vi "S Parameter Pre-Processing.vi"(6 "Username (\"\")":string, 7 "Fields In":T1[](array[typedef]), 8 "error in (no error)":errorcluster, 10 "Test Configuration (\"\")":string, 11 "Test_ID (\"\")":string) -> (0 "error out":errorcluster, 1 "Files Found?":bool, 2 "New Test Configuration":string, 3 "Dup Test_ID":string, 5 "Fields Out":T1[](array[typedef]))   [LabVIEW 2011]
uses:
  typedefs/Field Record.ctl
  typedefs/Field DataTypes.ctl
  typedefs/Field NextItem.ctl
  typedefs/Field System Fields.ctl
  TypeDefs/SP Limit Point.ctl
  LIB/S Parameter Version.vi
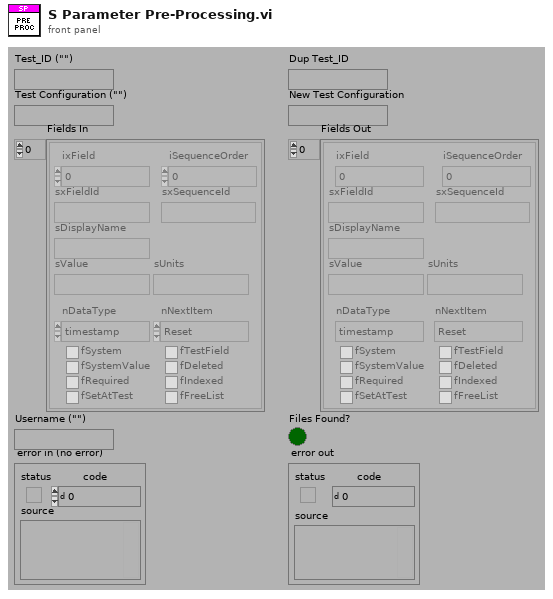
[diagram p1: front panel]
types:
  T1 = typedef "Field Record.ctl" = cluster{"ixField":i32, "iSequenceOrder":i32, "sxFieldId":string, "sxSequenceId":string, "sDisplayName":string, "sValue":string, "sUnits":string, "nDataType":T2, "nNextItem":T3, "fSystem":bool, "fSystemValue":bool, "fRequired":bool, "fSetAtTest":bool, "fTestField":bool, "fDeleted":bool, "fIndexed":bool, "fFreeList":bool}
  T2 = typedef "Field DataTypes.ctl" = enum32{"text", "numeric", "list", "timestamp", "boolean"}
  T3 = typedef "Field NextItem.ctl" = enum32{"Reset", "Retain", "Auto-Increment"}
  T4 = cluster{"Ref Limit":bool, "Ref Type":bool, "Model":bool, "Serial":bool, "Run Type":bool, "Run":bool, "Field":bool, "Field Value":bool}
  T5 = typedef "Field System Fields.ctl" = enum32{"Company", "End_Timestamp", "Model_Number", "Operator", "Serial_Number", "Start_Timestamp", "Step_Number", "Step_Tag", "Test_Run", "Test_Sequence", "Test_Station", "Test_Station_Name", "Test_Status", "Test_Type", "Test_Version", "Spartan_Version_Created", "Spartan_Version_Current"}
  T6 = typedef "SP Limit Point.ctl" = cluster{"Frequency":dbl, "Value":dbl, "X":dbl, "Y":dbl, "Connected":bool}
  T7 = typedef "SP Test Parameters.ctl" = cluster{"Stimulus":T8, "Measurement":T11, "De-Embed":T14, "Display":T17, "Limits":T24[], "Filter Limits":T28[]}
  T8 = typedef "SP Stimulus Parameters.ctl" = cluster{"Use Instrument Settings":bool, "Blank Frequencies":bool, "Sweep Type":enum32{"Linear", "Logarithmic", "List", "Power", "CW"}, "Sweep":cluster{"Fstart":dbl, "Fstop":dbl, "Units":T9, "Points":i32}, "Power (dBm)":dbl, "IFBW (Hz)":dbl, "Sweep Time (s)":dbl, "Calibration":T10}
  T9 = typedef "SP Frequency Units.ctl" = enum16{"Hz", "kHz", "MHz", "GHz", "Points"}
  T10 = typedef "SP Calibration State.ctl" = cluster{"State":bool, "String":string}
  T11 = typedef "SP Measurement.ctl" = cluster{"Auto Select":bool, "Data Source":enum16{"VNA", "Data File"}, "Ports":i8, "Parameters":T12[]}
  T12 = typedef "SP Parameters.ctl" = cluster{"Channel":i8, "Parameter":T13}
  T13 = typedef "SP Parameter.ctl" = cluster{"Stimulus Port":i8, "Response Port":i8}
  T14 = typedef "SP De-Embed.ctl" = cluster{"De-Embed":bool, "Adapters":T15[]}
  T15 = typedef "SP Adapter.ctl" = cluster{"Port":i8, "Order":i8, "Model Number":string, "Serial Number":string, "SP Data":T16, "Run Type":enum16{"Most Recent", "Run #", "Match Field"}, "Run":i32, "Field":string, "Field Value":string}
  T16 = typedef "SP Data.ctl" = cluster{"F0":dbl, "dF":dbl, "Data":cdb[][]}
  T17 = typedef "SP Display Parameters.ctl" = cluster{"Lock Control":bool, "Retain Settings":bool, "Formatted Data":bool, "Plot Orientation":enum32{"Single", "Dual", "Quad"}, "Plot Controls":T18[]}
  T18 = typedef "SP Display Plot Controls Cluster.ctl" = cluster{"Trace Orientation":enum32{"Overlay", "Split"}, "Frequency":cluster{"Change Frequency":bool, "Start":dbl, "Stop":dbl, "Units":T9}, "Markers":T19[], "Traces":T21[]}
  T19 = typedef "SP Marker Cluster.ctl" = cluster{"Type":T20, "Frequency (MHz)":dbl}
  T20 = typedef "SP Marker Type.ctl" = enum16{"Frequency", "Trace Maximum", "Trace Minimum", "Limit Maximum", "Limit Minimum"}
  T21 = typedef "SP Display Trace Controls.ctl" = cluster{"Trace On":bool, "Measure":i32, "Format":T22, "Autoscale":bool, "Reference":dbl, "\nRefUnit":string, "Position":dbl, "Scale":dbl, "ScaleUnit":string, "LimitOn":bool, "LimitFill":bool, "Display Data":T23, "Show Markers":bool, "SXX":string}
  T22 = typedef "SP Display Format.ctl" = i32
  T23 = typedef "SP Display Data.ctl" = u16
  T24 = typedef "SP Limit.ctl" = cluster{"Parameter":T13, "Format":T25, "Limit Type":T26, "Points":T6[], "Referential Limit":T27, "Limit #":i8}
  T25 = typedef "SP Format.ctl" = enum16{"Log Mag", "Lin Mag", "SWR", "Phase", "Expanded Phase", "Delay", "Insertion Loss", "Isolation", "Return Loss"}
  T26 = typedef "SP Limit Type.ctl" = enum16{"Upper", "Lower", "Delta", "Filter", "Referential"}
  T27 = typedef "Test Referential Limit.ctl" = cluster{"Ref Limit":bool, "Ref Type":enum16{"Current", "Specify"}, "Model":string, "Serial":string, "Run Type":enum16{"Most Recent", "Run #", "Match Field"}, "Run":i32, "Field":string, "Field Value":string}
  T28 = typedef "SP Filter.ctl" = cluster{"Limit #":i8, "Parameter":T13, "Format":T25, "Filter Type":T29, "Passband":T30, "Ripple":T32, "Attenuation Points":T33[], "Skirt Points":T35[]}
  T29 = typedef "SP Filter Type.ctl" = enum16{"Lowpass", "Highpass", "Bandpass", "Bandstop"}
  T30 = typedef "SP Filter Passband.ctl" = cluster{"Start/Center":dbl, "Stop/Span":dbl, "Units":T9, "Freq Format":T31, "Bandwidth Attn":dbl, "Passband Limit":bool}
  T31 = typedef "SP Frequency Format.ctl" = enum16{"Start/Stop", "Center/Span"}
  T32 = typedef "SP Filter Ripple.ctl" = cluster{"Ripple Limit":bool, "Window On":bool, "Ripple":dbl, "Window":dbl, "Units":T9}
  T33 = typedef "SP Attenuation Point.ctl" = cluster{"Attenuation":dbl, "Type":T34, "Lower":dbl, "Upper":dbl, "Units":T9}
  T34 = typedef "SP Attenuation Type.ctl" = enum16{"Center", "Lower", "Upper"}
  T35 = typedef "SP Skirt Rejection Point.ctl" = cluster{"Relative":bool, "Connect":bool, "Frequency":dbl, "Units":T9, "Attenuation":dbl, "Relative Loss":T36, "Relative Freq":dbl}
  T36 = typedef "SP Relative Loss.ctl" = enum16{"Calculated Center", "Passband Minimum", "Passband Maximum", "Passband Average", "Frequency"}
  T37 = cluster{"Parameter":cluster{"Stimulus Port":bool, "Response Port":bool}, "Format":bool, "Limit Type":bool, "Points":cluster{"Frequency":bool, "Value":bool, "X":bool, "Y":bool, "Connected":bool}[], "Referential Limit":cluster{"Ref Limit":bool, "Ref Type":bool, "Model":bool, "Serial":bool, "Run Type":bool, "Run":bool, "Field":bool, "Field Value":bool}, "Limit #":bool}
  T38 = typedef "Connection Refnum.ctl" = cluster{"Environment Handle":i32, "Connection Handle":i32}
  T39 = typedef "TDMS File.ctl" = cluster{"File Path":path, "Run Data":T40[], "Serial Number":string, "Model Number":string, "Test Type":string}
  T40 = typedef "TDMS Run.ctl" = cluster{"Channel Data":T41[], "Custom Fields":T1[], "Run ID":string}
  T41 = typedef "TDMS Channel (Sxx).ctl" = cluster{"Channel Name":string, "Waveform":dbl[], "Unit":string, "List value":string}
  T42 = typedef "OGAB Version.ctl" = cluster{"Version":string, "Build Number":u32, "Build Date/Time":dbl}
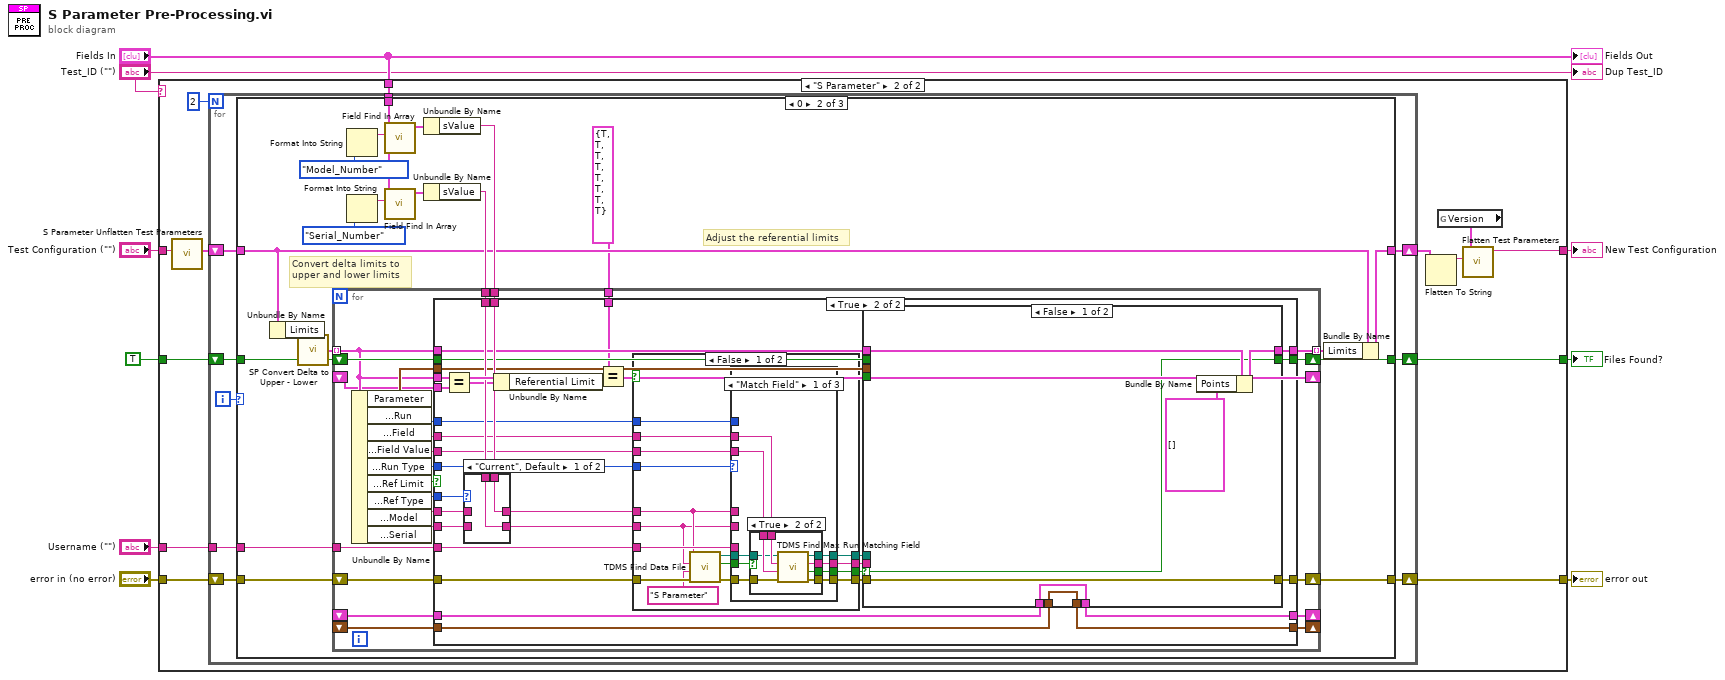
[diagram p0: block diagram]
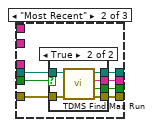
[diagram p6: hidden frame]
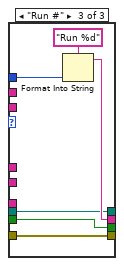
[diagram p8: hidden frame]
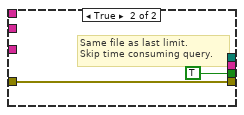
[diagram p9: hidden frame]
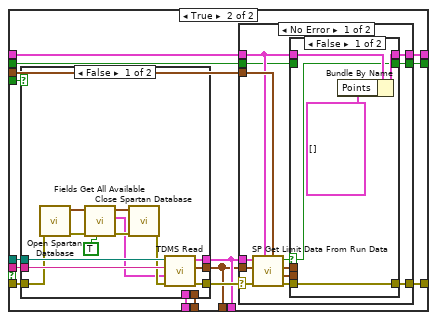
[diagram p10: hidden frame]
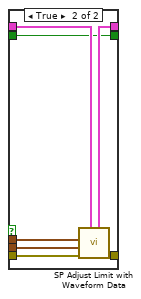
[diagram p11: hidden frame]
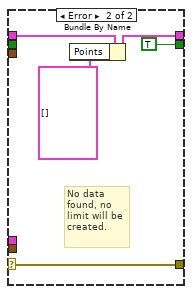
[diagram p12: hidden frame]
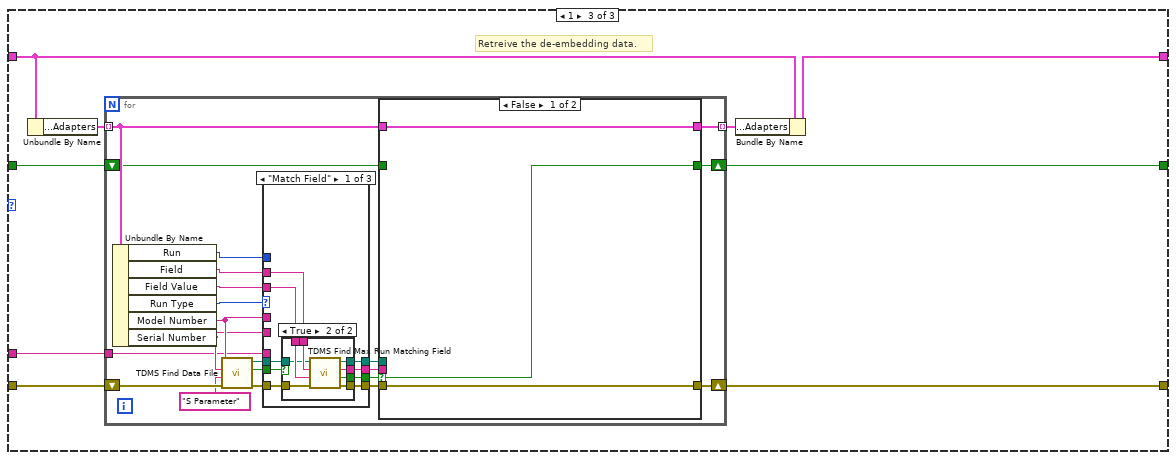
[diagram p15: hidden frame]
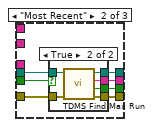
[diagram p17: hidden frame]
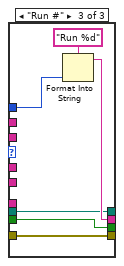
[diagram p19: hidden frame]
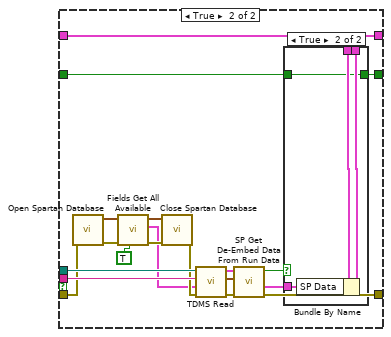
[diagram p20: hidden frame]
diagram:
  n1 = case shown="\"S Parameter\"" "Test_ID (\"\")" {
    tunnel: "Test Configuration (\"\")" -> [w12 w25]
    tunnel: [w12 w21] -> w8
    tunnel: "error in (no error)" -> [w11 w20]
    tunnel: [w11 w19] -> w5
    tunnel: "Fields In" -> [_ w18]
    tunnel: "Username (\"\")" -> [_ w17]
    tunnel: [w10 w14] -> w2
    tunnel: TRUE -> [w10 w13]
    frame Default {
    }
    frame "S Parameter" {
      n2 = call "S Parameter Unflatten Test Parameters.vi"("Parameter String"=w25) -> ("S Parameter Test Parameters"=w16:T7)  [unwired: 1 in, 9 out]
      n3 = for {
        N: 2 -> [_]
        tunnel: w18 -> [w31]
        tunnel: w17 -> [w30]
        shift-right: [w32] -> w19
        shift-left: w20 -> [w33]
        shift-right: [w34] -> w22
        shift-left: w16 -> [w29]
        shift-right: [w27] -> w14
        shift-left: w13 -> [w26]
        i -> [w28]
        n4 = case shown="0" w28 {
          tunnel: [w37 w57 w259] -> w34
          tunnel: w33 -> [w36 w56 w258]
          tunnel: [w36 w55 w257] -> w32
          tunnel: w31 -> [_ w48 _]
          tunnel: w30 -> [_ w45 w256]
          tunnel: w29 -> [w37 w44 w255]
          tunnel: [w35 w40 w251] -> w27
          tunnel: w26 -> [w35 w39 w252]
          frame Default {
          }
          frame 0 {
            # "Convert delta limits to\nupper and lower limits"
            # "Adjust the referential limits"
            n5 = Unbundle By Name(w44) -> ("Limits"=w42:T24[])
            n6 = call "SP Convert Delta to Upper - Lower.vi"("Limits"=w42) -> ("Converted Limits"=w41:T24[])  [unwired: 4 out]
            n7 = Format Into String(Field_System_Fields."Model_Number" ("System Field to Replace (Serial Number)")) -> (resulting string=w52:string)  [unwired: 3 in, 1 out]
            n8 = Format Into String(Field_System_Fields."Serial_Number" ("System Field to Replace (Serial Number)")) -> (resulting string=w51:string)  [unwired: 3 in, 1 out]
            n9 = call "Field Find In Array.vi"("FieldID or Display Name(\"\")"=w52, "Field Array"=w48) -> ("Field"=w54:T1)  [unwired: 1 in, 8 out]
            n10 = call "Field Find In Array.vi"("FieldID or Display Name(\"\")"=w51, "Field Array"=w48) -> ("Field"=w49:T1)  [unwired: 1 in, 8 out]
            n11 = Unbundle By Name(w54) -> ("sValue"=w47:string)
            n12 = Unbundle By Name(w49) -> ("sValue"=w46:string)
            n13 = for {
              tunnel: w41 -> [w64] mode=indexing
              tunnel: [w81] -> w43 mode=indexing
              shift-right: [w73] -> w55
              shift-left: w56 -> [w74]
              tunnel: w47 -> [w72]
              tunnel: w46 -> [w71]
              tunnel: w45 -> [w68]
              shift-right: [w66] -> w40
              shift-left: w39 -> [w65]
              shift-right: [w64] -> _
              shift-left: _ -> [w63]
              tunnel: T4 {"Ref Limit"=TRUE, "Ref Type"=TRUE, "Model"=TRUE, "Serial"=TRUE, "Run Type"=TRUE, "Run"=TRUE, "Field"=TRUE, "Field Value"=TRUE} ("Referential Limit") -> [w62]
              shift-right: [w61] -> _
              shift-left: _ -> [w58]
              shift-right: [w60] -> _
              shift-left: _ -> [w59]
              n14 = Unbundle By Name(w64) -> ("Parameter"=w67:T13, "Referential Limit.Run"=w69:i32, "Referential Limit.Field"=w75:string, "Referential Limit.Field Value"=w76:string, "Referential Limit.Run Type"=w77:enum16{"Most Recent", "Run #", "Match Field"}, "Referential Limit.Ref Limit"=w70:bool, "Referential Limit.Ref Type"=w78:enum16{"Current", "Specify"}, "Referential Limit.Model"=w79:string, "Referential Limit.Serial"=w80:string)
              n15 = case shown="True" w70 {
                tunnel: w64 -> [w85 w113]
                tunnel: [w85 w112] -> w81
                tunnel: w80 -> [_ w116]
                tunnel: w79 -> [_ w117]
                tunnel: w78 -> [_ w118]
                tunnel: w77 -> [_ w94]
                tunnel: w76 -> [_ w95]
                tunnel: w75 -> [_ w96]
                tunnel: w74 -> [w86 w90]
                tunnel: [w86 w111] -> w73
                tunnel: w67 -> [_ w110]
                tunnel: w72 -> [_ w115]
                tunnel: w71 -> [_ w114]
                tunnel: w69 -> [_ w98]
                tunnel: w68 -> [_ w91]
                tunnel: [w84 w109] -> w66
                tunnel: w65 -> [w84 w108]
                tunnel: w64 -> [_ w105]
                tunnel: w63 -> [_ w104]
                tunnel: w62 -> [_ w103]
                tunnel: [w83 w102] -> w61
                tunnel: [w82 w101] -> w60
                tunnel: w59 -> [w82 w100]
                tunnel: w58 -> [w83 w99]
                frame False {
                }
                frame True {
                  n16 = Equal?(x=w105, y=w104) -> (x = y?=w106:T37)
                  n17 = case shown="\"Current\", Default" w118 {
                    tunnel: w117 -> [_ w250]
                    tunnel: w116 -> [_ w249]
                    tunnel: [w248 w250] -> w93
                    tunnel: [w247 w249] -> w92
                    tunnel: w115 -> [w248 _]
                    tunnel: w114 -> [w247 _]
                    frame "Current", Default {
                    }
                    frame "Specify" {
                    }
                  }
                  n18 = Unbundle By Name(w106) -> ("Referential Limit"=w107:T4)
                  n19 = Equal?(x=w103, y=w107) -> (x = y?=w97:bool)
                  n20 = case shown="False" w97 {
                    tunnel: w94 -> [w134 _]
                    tunnel: w95 -> [w133 _]
                    tunnel: w96 -> [w132 _]
                    tunnel: w93 -> [w122 _]
                    tunnel: w92 -> [w121 _]
                    tunnel: [w131 _] -> w87
                    tunnel: w98 -> [w130 _]
                    tunnel: w91 -> [w129 _]
                    tunnel: [w128 w178] -> _
                    tunnel: w90 -> [w124 w178]
                    tunnel: [w127 _] -> w88
                    tunnel: [w126 TRUE ("Found?")] -> w89
                    frame False {
                      n21 = call "TDMS Find Data File.vi"("error in (no error)"=w124, "Test Type"="S Parameter" ("Value"), "Serial Number"=w121, "Model Number"=w122) -> ("error out"=w123:errorcluster, "Found?"=w119:bool, "TDMS Path"=w120:path)  [unwired: 5 in]
                      n22 = case shown="\"Match Field\"" w134 {
                        tunnel: w132 -> [w143 _ _]
                        tunnel: w133 -> [w142 _ _]
                        tunnel: w123 -> [w137 w157 w172]
                        tunnel: [w141 w161 w172] -> w128
                        tunnel: w122 -> [_ _ _]
                        tunnel: w121 -> [_ _ _]
                        tunnel: [w140 w160 w173] -> w127
                        tunnel: [w139 w159 w174] -> w131
                        tunnel: w130 -> [_ _ w175]
                        tunnel: w129 -> [_ _ _]
                        tunnel: [w138 w158 w171] -> w126
                        tunnel: w120 -> [w136 w156 w173]
                        tunnel: w119 -> [w135 w155 w171]
                        frame "Match Field" {
                          n23 = case shown="True" w135 {
                            selector: w135 -> [w144 _]
                            tunnel: w143 -> [_ w154]
                            tunnel: w142 -> [_ w153]
                            tunnel: w136 -> [w146 w152]
                            tunnel: w137 -> [w145 w151]
                            tunnel: [w145 w150] -> w141
                            tunnel: [w146 w149] -> w140
                            tunnel: [_ w148] -> w139
                            tunnel: [w144 w147] -> w138
                            frame False {
                            }
                            frame True {
                              n24 = call "TDMS Find Max Run Matching Field.vi"("error in (no error)"=w151, "Property Value"=w153, "Property Name"=w154, "TDMS File Path"=w152) -> ("error out"=w150:errorcluster, "Found?"=w147:bool, "Run ID"=w148:string, "TDMS File Path Out"=w149:path)  [unwired: 4 in]
                            }
                          }
                        }
                        frame "Most Recent" {
                          n25 = case shown="True" w155 {
                            selector: w155 -> [w162 _]
                            tunnel: w156 -> [w164 w170]
                            tunnel: w157 -> [w163 w169]
                            tunnel: [w163 w168] -> w161
                            tunnel: [w164 w167] -> w160
                            tunnel: [_ w166] -> w159
                            tunnel: [w162 w165] -> w158
                            frame False {
                            }
                            frame True {
                              n26 = call "TDMS Find Max Run.vi"("error in (no error)"=w169, "TDMS File Path"=w170) -> ("error out"=w168:errorcluster, "Found?"=w165:bool, "Run ID"=w166:string, "TDMS File Path Out"=w167:path)  [unwired: 6 in]
                            }
                          }
                        }
                        frame "Run #" {
                          n27 = Format Into String(format string="Run %d", w175) -> (resulting string=w174:string)  [unwired: 2 in, 1 out]
                        }
                      }
                    }
                    frame True {
                      # "Same file as last limit.\nSkip time consuming query."
                    }
                  }
                  n28 = case shown="False" w89 {
                    selector: w89 -> [w179 _]
                    tunnel: w113 -> [w185 w198]
                    tunnel: [w184 w197] -> w112
                    tunnel: [w182 w199] -> w111
                    tunnel: w110 -> [_ w200]
                    tunnel: w88 -> [_ w196]
                    tunnel: w87 -> [_ w195]
                    tunnel: w90 -> [w182 w192]
                    tunnel: [w179 w193] -> w109
                    tunnel: w108 -> [_ w194]
                    tunnel: w97 -> [_ w191]
                    tunnel: [w180 w189] -> w102
                    tunnel: [w181 w188] -> w101
                    tunnel: w100 -> [w181 w187]
                    tunnel: w99 -> [w180 w186]
                    frame False {
                      n29 = Bundle By Name(cluster=w185, "Points"=T6[] [] ("Lower")) -> (w184:T24)
                    }
                    frame True {
                      n30 = case shown="False" w191 {
                        tunnel: [w243 w246] -> w190
                        tunnel: [w242 w244] -> w189
                        tunnel: [w241 w245] -> w188
                        tunnel: w196 -> [w240 _]
                        tunnel: w195 -> [w239 _]
                        tunnel: w192 -> [w233 w246]
                        tunnel: w187 -> [_ w245]
                        tunnel: w186 -> [_ w244]
                        frame False {
                          n31 = call "Open Spartan Database.vi"("error in (no error)"=w233) -> ("error out"=w234:errorcluster, "Connection Refnum"=w235:T38)  [unwired: 9 in]
                          n32 = call "Fields Get All Available.vi"("Combine All? (f)"=TRUE, "error in (no error)"=w234, "Connection Refnum"=w235) -> ("error out"=w237:errorcluster, "System or ALL Combined Fields"=w231:T1[], "Connection Refnum"=w238:T38)  [unwired: 3 in, 3 out]
                          n33 = call "Close Spartan Database.vi"("error in (no error)"=w237, "Connection Refnum"=w238) -> ("error out"=w232:errorcluster)  [unwired: 9 in]
                          n34 = call "TDMS Read.vi"("error in (no error)"=w232, "System or ALL Combined Fields"=w231, "Run String"=w239, "TDM File Path"=w240) -> ("error out"=w243:errorcluster, "Run Waveforms"=w241:waveform(dbl)[], "File Information"=w242:T39)  [unwired: 3 in, 2 out]
                        }
                        frame True {
                          # "Same file as last limit.\nSkip time consuming read."
                        }
                      }
                      n35 = case shown="No Error" w190 {
                        selector: w190 -> [w201 w230]
                        tunnel: w200 -> [w213 _]
                        tunnel: [w210 w230] -> w199
                        tunnel: w198 -> [w208 w228]
                        tunnel: [w207 w227] -> w197
                        tunnel: w189 -> [w205 _]
                        tunnel: w188 -> [w204 _]
                        tunnel: w194 -> [w203 _]
                        tunnel: [w202 TRUE] -> w193
                        frame No Error {
                          n36 = call "SP Get Limit Data From Run Data.vi"("Parameter"=w213, "Limit"=w208, "error in (no error)"=w201, "Run Waveforms"=w204, "File Information"=w205) -> ("error out"=w212:errorcluster, "Data Waveform"=w206:waveform(dbl), "Frequency Waveform"=w209:waveform(dbl), "Found?"=w211:bool)  [unwired: 3 out]
                          n37 = case shown="False" w211 {
                            selector: w211 -> [w215 _]
                            tunnel: w212 -> [w214 w225]
                            tunnel: [w214 w224] -> w210
                            tunnel: w209 -> [_ w223]
                            tunnel: w208 -> [w216 w220]
                            tunnel: [w217 w221] -> w207
                            tunnel: w206 -> [_ w222]
                            tunnel: w203 -> [_ w219]
                            tunnel: [w215 w219] -> w202
                            frame False {
                              n38 = Bundle By Name(cluster=w216, "Points"=T6[] [] ("Lower")) -> (w217:T24)
                            }
                            frame True {
                              n39 = call "SP Adjust Limit with Waveform Data.vi"("Limit"=w220, "error in (no error)"=w225, "Data Waveform"=w222, "Frequency Waveform"=w223) -> ("error out"=w224:errorcluster, "Modified Limit"=w221:T24)  [unwired: 6 out]
                            }
                          }
                        }
                        frame Error {
                          # "No data\nfound, no\nlimit will be\ncreated."
                          n40 = Bundle By Name(cluster=w228, "Points"=T6[] [] ("Lower")) -> (w227:T24)
                        }
                      }
                    }
                  }
                }
              }
            }
            n41 = Bundle By Name(cluster=w44, "Limits"=w43) -> (w57:T7)
          }
          frame 1 {
            # "Retreive the de-embedding data."
            n42 = Unbundle By Name(w255) -> ("De-Embed.Adapters"=w254:T15[])
            n43 = for {
              tunnel: w254 -> [w280] mode=indexing
              tunnel: [w279] -> w253 mode=indexing
              shift-right: [w278] -> w257
              shift-left: w258 -> [w275]
              tunnel: w256 -> [w268]
              shift-right: [w276] -> w251
              shift-left: w252 -> [w277]
              n44 = Unbundle By Name(w280) -> ("Run"=w274:i32, "Field"=w273:string, "Field Value"=w272:string, "Run Type"=w271:enum16{"Most Recent", "Run #", "Match Field"}, "Model Number"=w270:string, "Serial Number"=w269:string)
              n45 = call "TDMS Find Data File.vi"("error in (no error)"=w275, "Test Type"="S Parameter" ("Value"), "Serial Number"=w269, "Model Number"=w270) -> ("error out"=w262:errorcluster, "Found?"=w260:bool, "TDMS Path"=w261:path)  [unwired: 5 in]
              n46 = case shown="\"Match Field\"" w271 {
                tunnel: w273 -> [w289 _ _]
                tunnel: w272 -> [w288 _ _]
                tunnel: w262 -> [w283 w303 w318]
                tunnel: [w287 w307 w318] -> w267
                tunnel: w270 -> [_ _ _]
                tunnel: w269 -> [_ _ _]
                tunnel: [w286 w306 w319] -> w265
                tunnel: [w285 w305 w320] -> w264
                tunnel: w274 -> [_ _ w321]
                tunnel: w268 -> [_ _ _]
                tunnel: [w284 w304 w317] -> w266
                tunnel: w261 -> [w282 w302 w319]
                tunnel: w260 -> [w281 w301 w317]
                frame "Match Field" {
                  n47 = case shown="True" w281 {
                    selector: w281 -> [w290 _]
                    tunnel: w289 -> [_ w300]
                    tunnel: w288 -> [_ w299]
                    tunnel: w282 -> [w292 w298]
                    tunnel: w283 -> [w291 w297]
                    tunnel: [w291 w296] -> w287
                    tunnel: [w292 w295] -> w286
                    tunnel: [_ w294] -> w285
                    tunnel: [w290 w293] -> w284
                    frame False {
                    }
                    frame True {
                      n48 = call "TDMS Find Max Run Matching Field.vi"("error in (no error)"=w297, "Property Value"=w299, "Property Name"=w300, "TDMS File Path"=w298) -> ("error out"=w296:errorcluster, "Found?"=w293:bool, "Run ID"=w294:string, "TDMS File Path Out"=w295:path)  [unwired: 4 in]
                    }
                  }
                }
                frame "Most Recent" {
                  n49 = case shown="True" w301 {
                    selector: w301 -> [w308 _]
                    tunnel: w302 -> [w310 w316]
                    tunnel: w303 -> [w309 w315]
                    tunnel: [w309 w314] -> w307
                    tunnel: [w310 w313] -> w306
                    tunnel: [_ w312] -> w305
                    tunnel: [w308 w311] -> w304
                    frame False {
                    }
                    frame True {
                      n50 = call "TDMS Find Max Run.vi"("error in (no error)"=w315, "TDMS File Path"=w316) -> ("error out"=w314:errorcluster, "Found?"=w311:bool, "Run ID"=w312:string, "TDMS File Path Out"=w313:path)  [unwired: 6 in]
                    }
                  }
                }
                frame "Run #" {
                  n51 = Format Into String(format string="Run %d", w321) -> (resulting string=w320:string)  [unwired: 2 in, 1 out]
                }
              }
              n52 = case shown="False" w266 {
                selector: w266 -> [w323 _]
                tunnel: w280 -> [w324 w344]
                tunnel: [w324 w343] -> w279
                tunnel: [w325 w337] -> w278
                tunnel: w265 -> [_ w338]
                tunnel: w267 -> [w325 w328]
                tunnel: w277 -> [_ w336]
                tunnel: [w323 w335] -> w276
                tunnel: w264 -> [_ w334]
                frame False {
                }
                frame True {
                  n53 = call "Open Spartan Database.vi"("error in (no error)"=w328) -> ("error out"=w329:errorcluster, "Connection Refnum"=w330:T38)  [unwired: 9 in]
                  n54 = call "Fields Get All Available.vi"("Combine All? (f)"=TRUE, "error in (no error)"=w329, "Connection Refnum"=w330) -> ("error out"=w332:errorcluster, "System or ALL Combined Fields"=w326:T1[], "Connection Refnum"=w333:T38)  [unwired: 3 in, 3 out]
                  n55 = call "Close Spartan Database.vi"("error in (no error)"=w332, "Connection Refnum"=w333) -> ("error out"=w327:errorcluster)  [unwired: 9 in]
                  n56 = call "TDMS Read.vi"("error in (no error)"=w327, "System or ALL Combined Fields"=w326, "Run String"=w334, "TDM File Path"=w338) -> ("error out"=w341:errorcluster, "Run Waveforms"=w339:waveform(dbl)[], "File Information"=w340:T39)  [unwired: 3 in, 2 out]
                  n57 = call "SP Get De-Embed Data From Run Data.vi"("error in (no error)"=w341, "Run Waveforms"=w339, "File Information"=w340) -> ("error out"=w337:errorcluster, "SP Data"=w342:T16, "Valid?"=w345:bool)  [unwired: 1 in, 5 out]
                  n58 = case shown="True" w345 {
                    tunnel: w344 -> [w347 w351]
                    tunnel: [w347 w350] -> w343
                    tunnel: w342 -> [_ w349]
                    tunnel: [FALSE w348] -> w335
                    tunnel: w336 -> [_ w348]
                    frame False {
                    }
                    frame True {
                      n59 = Bundle By Name(cluster=w351, "SP Data"=w349) -> (w350:T15)
                    }
                  }
                }
              }
            }
            n60 = Bundle By Name(cluster=w255, "De-Embed.Adapters"=w253) -> (w259:T7)
          }
        }
      }
      n61 = Flatten To String(anything=w22) -> (data string=w24:string)  [unwired: 1 in, 4 out]
      n62 = global read "S Parameter Version.vi" "Version"() -> (w23:T42)
      n63 = call "Flatten Test Parameters.vi"("Flattened Test Parameters (\"\")"=w24, "Test Version"=w23) -> ("Flattened Test Parameters with Version"=w21:string)  [unwired: 1 in, 4 out]
    }
  }
  "error out" <- w5
  "New Test Configuration" <- w8
  "Files Found?" <- w2
  "Dup Test_ID" <- "Test_ID (\"\")"
  "Fields Out" <- "Fields In"
